vi "AD2Digital Signal.vi"(10 "通道数":i32, 11 "AD":i16[](array[numeric])) -> (2 "CH2":dbl[](array[numeric]), 3 "CH1":dbl[](array[numeric]))   [LabVIEW 2015, in "DAQ.lvlib"]
uses:
  DAQ.lvlib
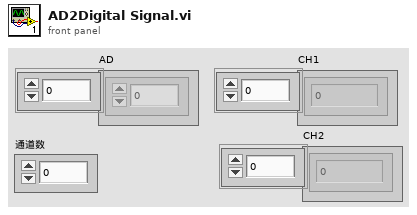
[diagram p1: front panel]
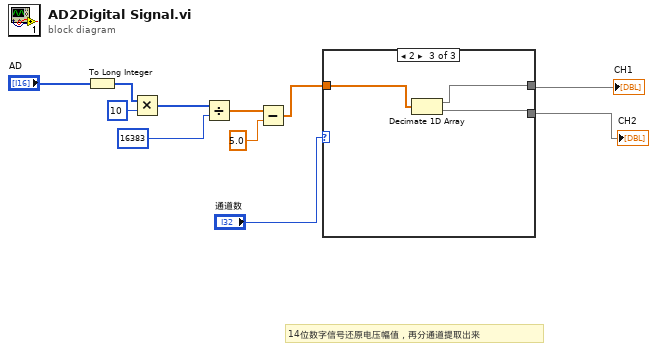
[diagram p0: block diagram]
diagram:
  # "14位数字信号还原电压幅值，再分通道提取出来"
  n1 = To Long Integer(number="AD") -> (32bit integer=w7:i32[])
  n2 = Multiply(x=w7, y=10) -> (x*y=w9:i32[])
  n3 = Divide(x=w9, y=16383) -> (x/y=w10:dbl[])
  n4 = Subtract(x=w10, y=5.0) -> (x-y=w5:dbl[])
  n5 = case shown="2" "通道数" {
    tunnel: w5 -> [_ w12 w15]
    tunnel: [_ w12 w14] -> w2
    tunnel: [_ _ w13] -> w1
    frame 0, Default {
    }
    frame 1 {
    }
    frame 2 {
      n6 = Decimate 1D Array(w15) -> (w14:dbl[], w13:dbl[])
    }
  }
  "CH1" <- w2
  "CH2" <- w1
